vi "Test Gmail Auth.vi"() -> ()   [LabVIEW 2020]
uses:
  Gmail API/Mail Address.ctl
  Gmail API/Gmail/Gmail.lvclass
  Gmail API/OAuth2/OAuth2.lvclass
  C:/Program Files (x86)/National Instruments/LabVIEW 2020/vi.lib/IlluminatedG/IG HTTP Utils/OAuth2/OAuth2/OAuth2.lvclass
  Gmail API/Gmail/Add To.vi
  Gmail API/Gmail/Set Subject.vi
  Gmail API/Gmail/Set Content-Type.vi
  Gmail API/Gmail/Set Body.vi
  <vilib>/IlluminatedG/IG HTTP Utils/OAuth2/Client/Client.lvclass
  <vilib>/IlluminatedG/IG HTTP Utils/OAuth2/OAuth2/OAuth2.lvclass
  <vilib>/IlluminatedG/IG HTTP Utils/OAuth2/Async Authorization/Async Authorization.lvclass
  Gmail API/Gmail API.lvlib
panel:
  in  "Name":string
  in  "Content-Type":string
  in  "Body":string
  in  "Subject":string
  in  "Email":string
  in  "From Account (Prompt)":string
  in  "Secret":string
  in  "ID":string
  out "error out":errorcluster
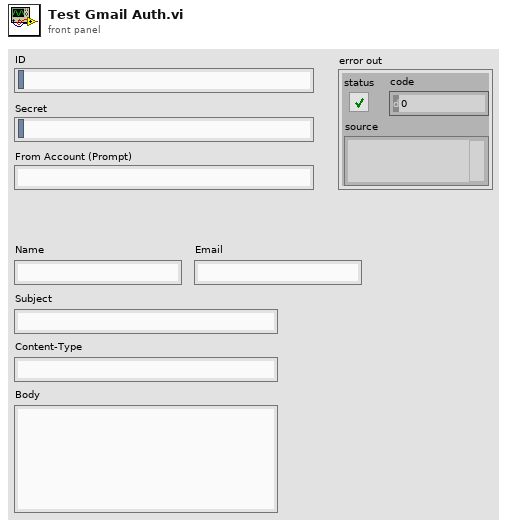
[diagram p1: front panel]
types:
  T1 = typedef "Gmail API.lvlib/Mail Address.ctl" = cluster{"Name":string, "Email":string}
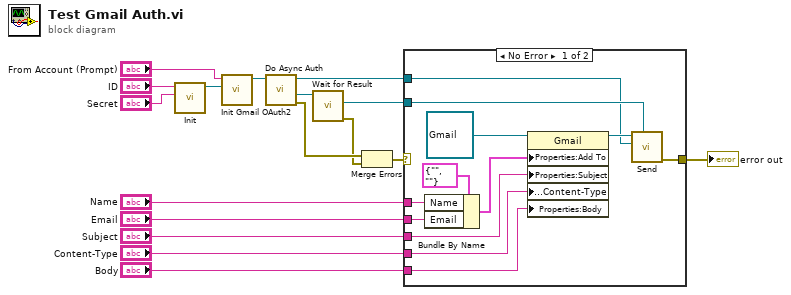
[diagram p0: block diagram]
diagram:
  n1 = call <vilib>:"Init.vi"("Secret"="Secret", "ID"="ID") -> ("Client out"=w17:refnum<class "Client.lvclass">)  [unwired: 9 in]
  n2 = call "Init Gmail OAuth2.vi"("Client"=w17, "Account (Prompt)"="From Account (Prompt)") -> ("OAuth2 out"=w14:refnum<class "OAuth2.lvclass">)  [unwired: 9 in]
  n3 = call <vilib>:"Do Async Auth.vi"("OAuth2 in"=w14) -> ("error out"=w12:errorcluster, "Async Authentication"=w13:refnum<class "Async Authorization.lvclass">, "OAuth2 out"=w7:refnum<class "OAuth2.lvclass">)  [unwired: 8 in]
  n4 = call <vilib>:"Wait for Result.vi"("Async Authorization in"=w13) -> ("error out"=w11:errorcluster, "Authorization"=w8:refnum<class "Authorization.lvclass">)  [unwired: 8 in, 1 out]
  n5 = Merge Errors(w12, w11) -> (w9:errorcluster)
  n6 = case shown="No Error" w9 {
    selector: w9 -> [_ w30]
    tunnel: w8 -> [w20 _]
    tunnel: w7 -> [w19 _]
    tunnel: "Email" -> [w27 _]
    tunnel: "Subject" -> [w25 _]
    tunnel: "Content-Type" -> [w24 _]
    tunnel: "Body" -> [w23 _]
    tunnel: "Name" -> [w28 _]
    tunnel: [w18 w30] -> w1
    frame No Error {
      n7 = Bundle By Name(cluster=T1 {"Name"="", "Email"=""} ("Mail Address"), "Name"=w28, "Email"=w27) -> (w26:T1)
      n8 = property class="Gmail"(reference=refnum<class "Gmail.lvclass"> refnum, "Properties:Add To"=w26, "Properties:Subject"=w25, "Properties:Content-Type"=w24, "Properties:Body"=w23) -> (reference out=w21:refnum<class "Gmail.lvclass">)  [unwired: 1 in, 1 out]
      n9 = call "Send.vi"("Authorization in"=w20, "Google OAuth"=w19, "Gmail in"=w21) -> ("error out"=w18:errorcluster)  [unwired: 6 in, 2 out]
    }
    frame Error {
    }
  }
  "error out" <- w1
